vi "Snapshot Blob.vi"(8 "error in (no error)":errorcluster, 9 "Blob":string, 10 "Container":string, 11 "Azure Session in":refnum<class "Session.lvclass">) -> (0 "error out":errorcluster, 2 "Snapshot":string, 3 "Azure Session out":refnum<class "Session.lvclass">)   [LabVIEW 2015, in "NI_Azure_Blob.lvlib"]
doc: "Creates a read-only snapshot of a blob."
uses:
  NI_Azure_Blob.lvlib
  Core/Session/Session.lvclass
  Core/Name Value Pair.ctl
  Core/Session/Session.lvclass/Session.ctl
  Core/Session/Write Request Parameters.vi
  Core/Session/Write URL Suffix.vi
  Core/Session/Write HTTP Verb.vi
  Core/NI_Azure_Core.lvlib
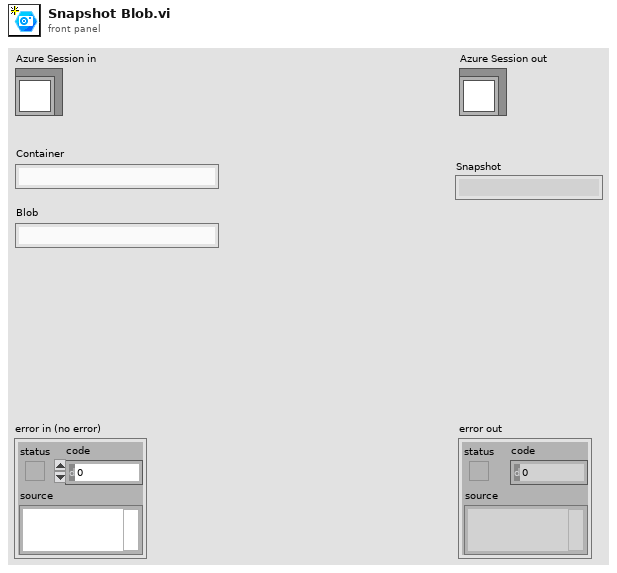
[diagram p1: front panel]
types:
  T1 = typedef "NI_Azure_Core.lvlib/Name Value Pair.ctl" = cluster{"name":string, "value":string}
  T2 = typedef "NI_Azure_Core.lvlib/Response.ctl" = cluster{"Headers":string, "Body":string}
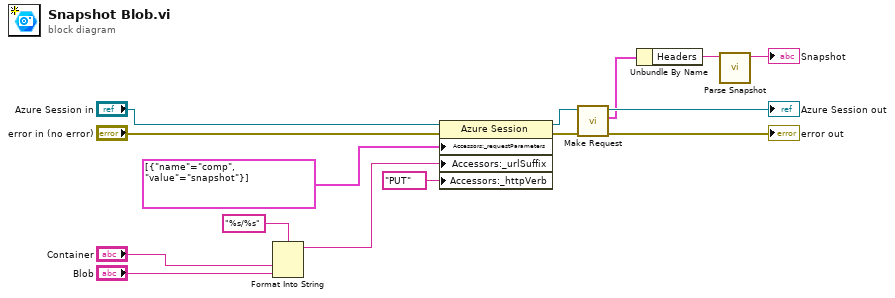
[diagram p0: block diagram]
diagram:
  n1 = Format Into String(format string="%s/%s", "Container", "Blob") -> (resulting string=w2:string)  [unwired: 2 in, 1 out]
  n2 = property class="Azure Session"(reference="Azure Session in", error in="error in (no error)", "Accessors:_requestParameters"=T1[] [{"name"="comp", "value"="snapshot"}] ("request parameters"), "Accessors:_urlSuffix"=w2, "Accessors:_httpVerb"="PUT" ("HTTP-Verb")) -> (reference out=w4:refnum<class "Session.lvclass">, error out=w6:errorcluster)
  n3 = call "Make Request.vi"("error in (no error)"=w6, "Session in"=w4) -> ("error out"=→"error out":errorcluster, "Response"=w7:T2, "Session out"=→"Azure Session out":refnum<class "Session.lvclass">)  [unwired: 7 in]
  n4 = Unbundle By Name(w7) -> ("Headers"=w8:string)
  n5 = call "Parse Snapshot.vi"("String"=w8) -> ("Date time"=→"Snapshot":string)  [unwired: 10 in]
